vi "Delacor_lib_QMH_Get Message Queue.vi"(8 "error in":errorcluster, 11 "Message Queue in":refnum<class "JQMH_Message Queue.lvclass">) -> (0 "error out":errorcluster, 2 "Message Queue":refnum<queue>, 3 "Message Queue out":refnum<class "JQMH_Message Queue.lvclass">)   [LabVIEW 2024, in "JQMH_Message Queue.lvclass"]
doc: "____\nDQMH Framework: Palette 7.1.0.1503\nCopyright (c) 2025, DQMH Consortium"
uses:
  JQMH_Message Queue.lvclass
  Delacor_lib_QMH_Message--cluster.ctl
  JQMH_Message Queue.lvclass/JQMH_Message Queue.ctl
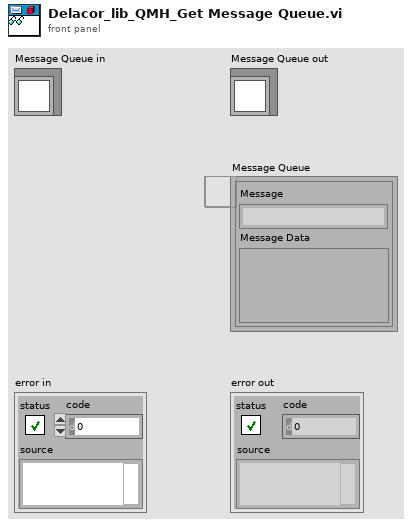
[diagram p1: front panel]
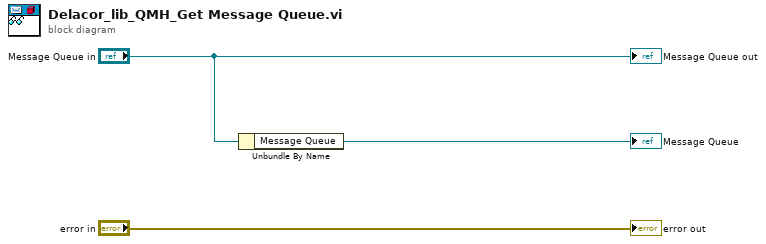
[diagram p0: block diagram]
diagram:
  n1 = Unbundle By Name("Message Queue in") -> ("Message Queue"=→"Message Queue":refnum<queue>)
  "error out" <- "error in"
  "Message Queue out" <- "Message Queue in"
